vi "Configure Client.vi"(8 "error in (no error)":errorcluster, 10 "Client in":refnum<class "Connection.lvclass">, 11 "Resource in":refnum<class "Resource.lvclass">) -> (0 "error out":errorcluster, 2 "Client":refnum<class "Connection.lvclass">, 3 "Resource out":refnum<class "Resource.lvclass">)   [LabVIEW 2020, in "PicoG-Core.lvlib" / "Resource.lvclass"]
uses:
  Resource.lvclass
  Resource.lvclass/Resource.ctl
  <vilib>/IlluminatedG/lv-stream/Connection/Connection.lvclass
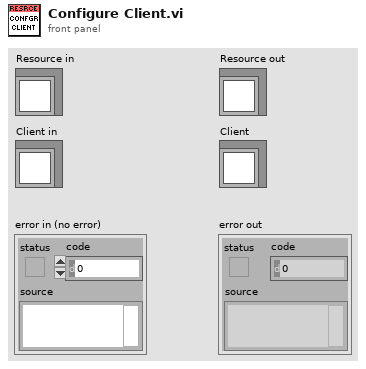
[diagram p1: front panel]
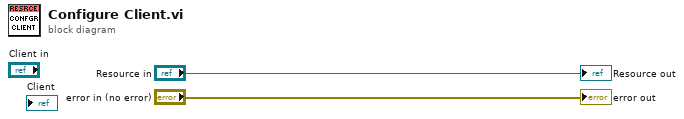
[diagram p0: block diagram]
diagram:
  "error out" <- "error in (no error)"
  "Resource out" <- "Resource in"
